vi "setModbus.vi"(10 "Modbus":refnum<class "Modbus.lvclass">, 11 "Mockbus in":refnum<class "Mockbus.lvclass">) -> (3 "Mockbus out":refnum<class "Mockbus.lvclass">)   [LabVIEW 2015, in "RTMockbus.lvlib" / "Mockbus.lvclass"]
uses:
  Mockbus.lvclass
  Common_RT_Modbus/Modbus/Modbus.lvclass
  Mockbus.lvclass/Mockbus.ctl
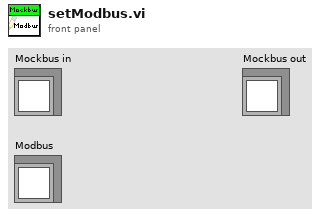
[diagram p1: front panel]
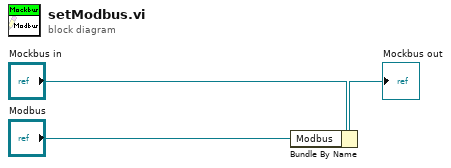
[diagram p0: block diagram]
diagram:
  n1 = Bundle By Name(cluster="Mockbus in", "Modbus"="Modbus") -> (→"Mockbus out":refnum<class "Mockbus.lvclass">)
